vi "Write.vi"(8 "error in (no error)":errorcluster, 10 "Log Data":T1={"Time"=timestamp(0 s since 1904-01-01), "Level"=enum."INFO", "Logger"="", "Message"="", "Arguments"=[]} {"Time" format="%<%x %.3X>T"}, 11 "Sink-Console in":refnum<class "Sink-Console.lvclass">) -> (0 "error out":errorcluster, 3 "Sink-Console out":refnum<class "Sink-Console.lvclass">)   [LabVIEW 2019, in "TSC Event Logger.lvlib" / "Sink-Console.lvclass"]
uses:
  Sink-Console.lvclass
  C:/Development/Reuse-libraries/Event Logger/Log Sinks/Log Sinks.lvclass
  Log Data.ctl
  Log/Event Level.ctl
  Sink-Console.lvclass/Sink-Console.ctl
  Log Sinks.lvclass
  TSC Event Logger.lvlib
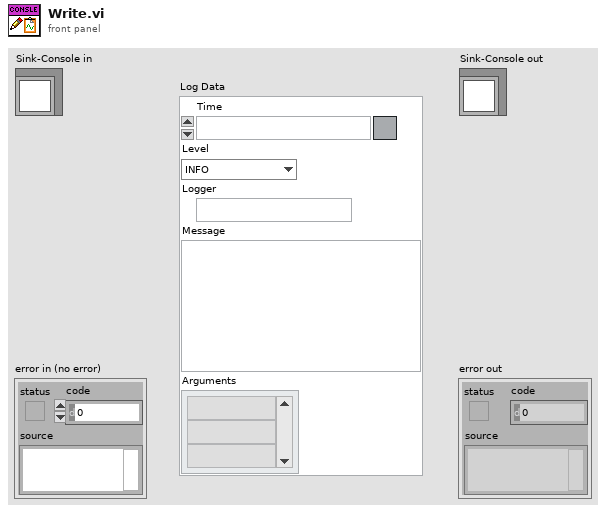
[diagram p1: front panel]
types:
  T1 = typedef "TSC Event Logger.lvlib/Log Data.ctl" = cluster{"Time":timestamp, "Level":T2, "Logger":string, "Message":string, "Arguments":string[]}
  T2 = typedef "TSC Event Logger.lvlib/Event Level.ctl" = enum16{"OFF", "TRACE", "DEBUG", "INFO", "WARN", "ERROR", "FATAL"}
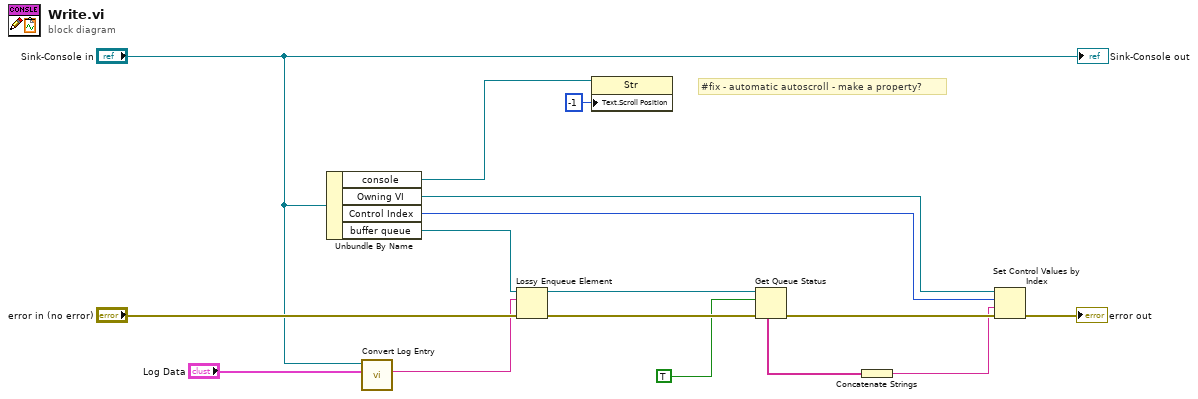
[diagram p0: block diagram]
diagram:
  # "#fix - automatic autoscroll - make a property?"
  n1 = Unbundle By Name("Sink-Console in") -> ("console"=w12:refnum<vi>, "Owning VI"=w14:refnum<vi>, "Control Index"=w13:i32, "buffer queue"=w9:refnum<queue>)
  n2 = call "Convert Log Entry.vi"("Log Data"="Log Data", "Log Sink in"="Sink-Console in") -> ("Log Entry"=w1:string)  [unwired: 9 in]
  n3 = Lossy Enqueue Element(queue=w9, element=w1, error in (no error)="error in (no error)") -> (queue out=w7:refnum<queue>, error out=w10:errorcluster)  [unwired: 2 out]
  n4 = property class="Str"(reference=w12, "Text.Scroll Position"=-1) -> ()  [unwired: 1 in, 2 out]
  n5 = Get Queue Status(queue=w7, return elements? (F)=TRUE, error in (no error)=w10) -> (error out=w8:errorcluster, elements=w6:string[])  [unwired: 6 out]
  n6 = Concatenate Strings(w6) -> (w5:string)
  n7 = Set Control Values by Index(0:w14, 1:w13, 2:w5, 3:w8) -> (11:→"error out":errorcluster)
  "Sink-Console out" <- "Sink-Console in"
